vi "05Foot_StoreFootfall.vi"(8 "error in (no error)":errorcluster, 10 "FootIn":string, 11 "Enum":T1(ring)) -> (0 "error out":errorcluster, 3 "FootOut":string)   [LabVIEW 2020]
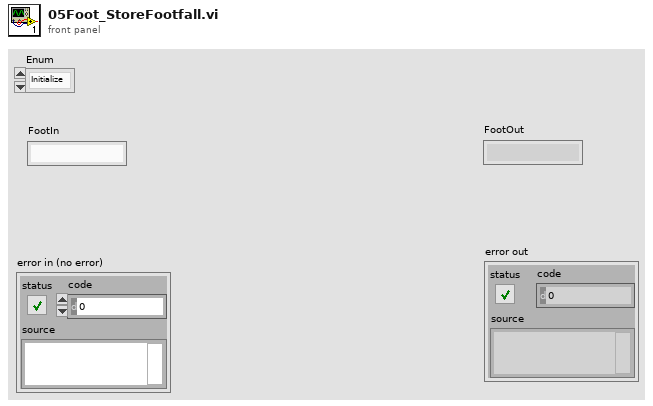
[diagram p1: front panel]
types:
  T1 = enum16{"Initialize", "FootReceive", "FootDisplay"}
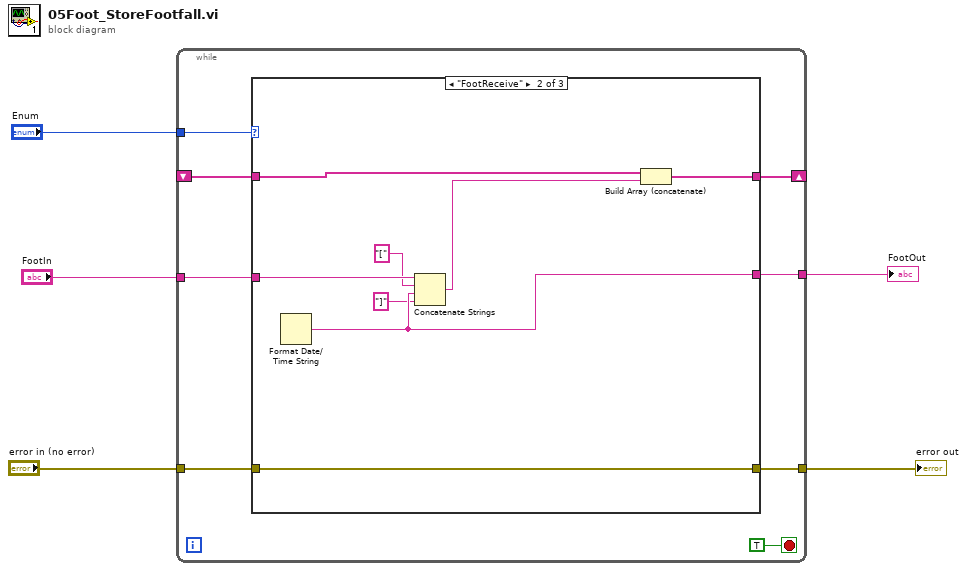
[diagram p0: block diagram]
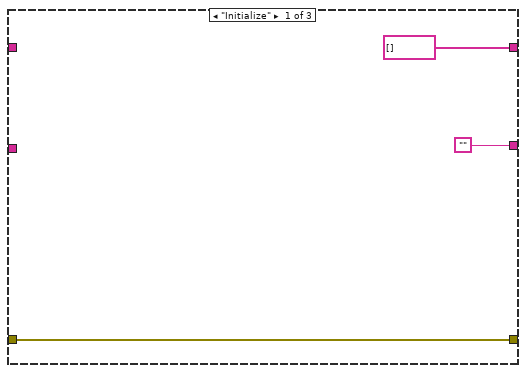
[diagram p2: hidden frame]
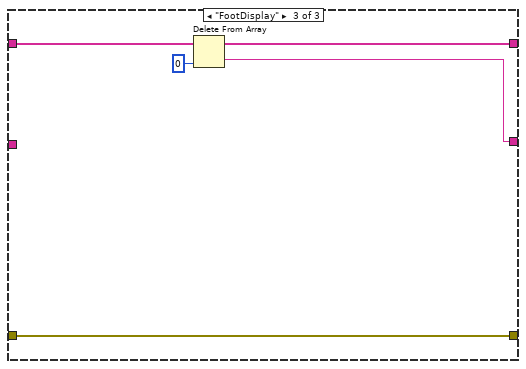
[diagram p3: hidden frame]
diagram:
  n1 = while {
    tunnel: "Enum" -> [w13]
    tunnel: "error in (no error)" -> [w12]
    tunnel: [w11] -> w3
    tunnel: "FootIn" -> [w10]
    shift-right: [w9] -> _
    shift-left: _ -> [w8]
    tunnel: [w7] -> w1
    stop <- TRUE stop-if-true
    n2 = case shown="\"FootReceive\"" w13 {
      tunnel: w12 -> [w16 w22 w29]
      tunnel: [w16 w22 w29] -> w11
      tunnel: w10 -> [_ w21 _]
      tunnel: [string[] [] w23 w26] -> w9
      tunnel: w8 -> [_ w24 w28]
      tunnel: ["" w18 w25] -> w7
      frame "Initialize" {
      }
      frame "FootReceive" {
        n3 = Format Date/Time String() -> (date/time string=w18:string)  [unwired: 3 in]
        n4 = Concatenate Strings(w21, "[" ("string"), w18, "]" ("string")) -> (w20:string)
        n5 = Build Array (concatenate)(w24, w20) -> (w23:string[])
      }
      frame "FootDisplay" {
        n6 = Delete From Array(array=w28, index=0) -> (deleted portion=w25:string, array with subset deleted=w26:string[])  [unwired: 1 in]
      }
    }
  }
  "error out" <- w3
  "FootOut" <- w1
